vi "生成CODMn data (子VI).vi"() -> (3 "data":T1)   [LabVIEW 2016, in "斯坦道CODMn.lvlib"]
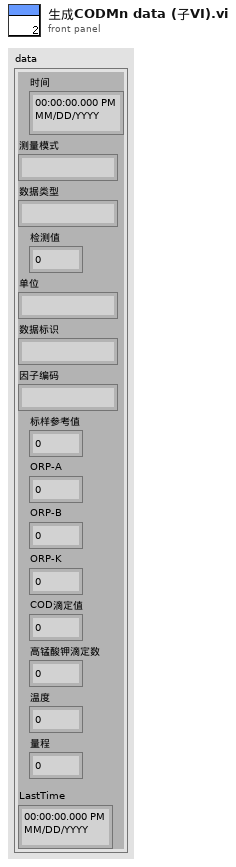
[diagram p1: front panel]
types:
  T1 = cluster{"时间":timestamp, "测量模式":string, "数据类型":string, "检测值":sgl, "单位":string, "数据标识":string, "因子编码":string, "标样参考值":sgl, "ORP-A":sgl, "ORP-B":sgl, "ORP-K":sgl, "COD滴定值":sgl, "高锰酸钾滴定数":sgl, "温度":sgl, "量程":sgl, "LastTime":timestamp}
  T2 = cluster{"运行模式":enum16{"维护模式", "常规模式", "应急模式", "质控模式"}}
  T3 = cluster{"测量量程":dbl, "测量精度":dbl, "测量间隔":dbl, "消解温度":dbl, "消解时长":dbl, "空白校准时间":timestamp, "曲线截距":dbl, "曲线斜率":dbl, "测量检出限":dbl, "测量信号值":dbl, "线性相关系数":dbl, "二次多项式系数":dbl, "标样校准时间":timestamp, "单位":u16}
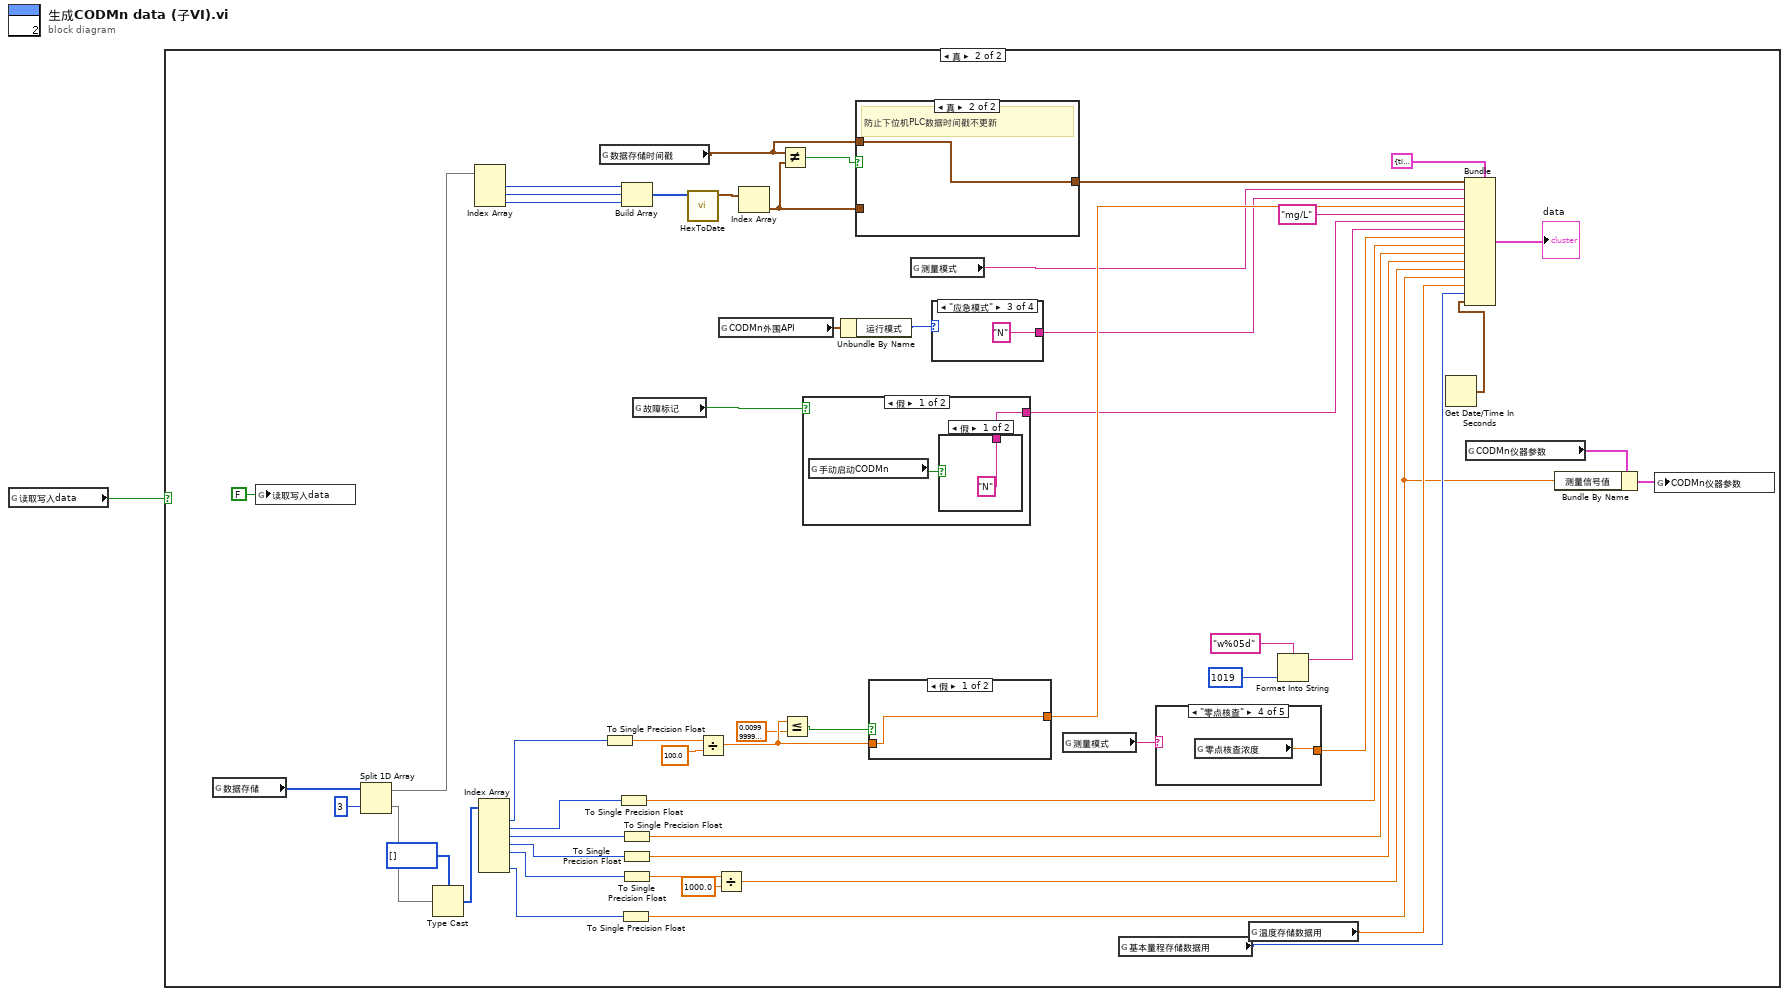
[diagram p0: block diagram]
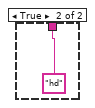
[diagram p4: hidden frame]
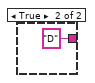
[diagram p5: hidden frame]
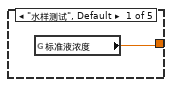
[diagram p6: hidden frame]
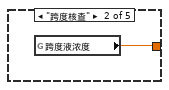
[diagram p7: hidden frame]
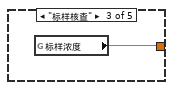
[diagram p8: hidden frame]
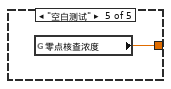
[diagram p9: hidden frame]
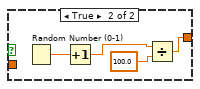
[diagram p10: hidden frame]
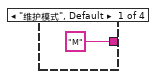
[diagram p11: hidden frame]
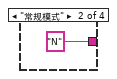
[diagram p12: hidden frame]
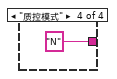
[diagram p13: hidden frame]
diagram:
  n1 = global read "COD内部交互全局.vi" "读取写入data"() -> (w1:bool)
  n2 = case shown="真" w1 {
    frame False {
    }
    frame True {
      n3 = global read "COD内部交互全局.vi" "数据存储"() -> (w7:u16[])
      n4 = global write "COD内部交互全局.vi" "读取写入data"(FALSE ("读取写入data")) -> ()
      n5 = Split 1D Array(array=w7, index=3 ("索引")) -> (first subarray=w15:u16[], second subarray=w6:u16[])
      n6 = Type Cast(type=i16[] [], x=w6) -> (*(type *) &x=w5:i16[])
      n7 = Index Array(array=w15) -> (element #1=w17:u16, element #2=w18:u16, element #3=w19:u16)  [unwired: 3 in]
      n8 = Index Array(array=w5) -> (element #1=w42:i16, element #2=w21:i16, element #3=w22:i16, element #4=w23:i16, element #5=w24:i16, element #7=w52:i16)  [unwired: 7 in, 1 out]
      n9 = global read "COD内部交互全局.vi" "数据存储时间戳"() -> (w53:timestamp)
      n10 = To Single Precision Float(number=w42) -> (single precision float=w40:sgl)
      n11 = To Single Precision Float(number=w21) -> (single precision float=w33:sgl)
      n12 = To Single Precision Float(number=w52) -> (single precision float=w2:sgl)
      n13 = Build Array(w17, w18, w19) -> (w20:u16[])
      n14 = To Single Precision Float(number=w22) -> (single precision float=w32:sgl)
      n15 = To Single Precision Float(number=w23) -> (single precision float=w31:sgl)
      n16 = To Single Precision Float(number=w24) -> (single precision float=w27:sgl)
      n17 = global read "COD内部交互全局.vi" "故障标记"() -> (w55:bool)
      n18 = call "HexToDate.vi"("数组"=w20) -> ("DATE"=w16:timestamp[])  [unwired: 10 in]
      n19 = Divide(x=w40, y=sgl 100.0) -> (x/y=w41:sgl)
      n20 = Divide(x=w27, y=sgl 1000.0) -> (x/y=w30:sgl)
      n21 = global read "CODMN外部API.vi" "CODMn外围API"() -> (w45:T2)
      n22 = Index Array(array=w16) -> (element=w48:timestamp)  [unwired: 1 in]
      n23 = Not Equal?(x=w53, y=w48) -> (x != y?=w49:bool)
      n24 = Less Or Equal?(x=w41, y=sgl 0.01) -> (x <= y?=w39:bool)
      n25 = case shown="假" w55 {
        tunnel: [w59 "D" ("数据标识")] -> w35
        frame False {
          n26 = global read "CODMN外部API.vi" "手动启动CODMn"() -> (w58:bool)
          n27 = case shown="假" w58 {
            tunnel: ["N" ("数据标识") "hd" ("数据标识")] -> w59
            frame False {
            }
            frame True {
            }
          }
        }
        frame True {
        }
      }
      n28 = Unbundle By Name(w45) -> ("运行模式"=w46:enum16{"维护模式", "常规模式", "应急模式", "质控模式"})
      n29 = case "条件结构" shown="真" w49 {
        tunnel: w48 -> [w56 _]
        tunnel: w53 -> [_ w57]
        tunnel: [w56 w57] -> w50
        frame False {
        }
        frame True {
          # "防止下位机PLC数据时间戳不更新"
        }
      }
      n30 = case shown="假" w39 {
        tunnel: [w68 w69] -> w51
        tunnel: w41 -> [w68 _]
        frame False {
        }
        frame True {
          n31 = Random Number (0-1)() -> (number: 0 to 1=w72:dbl)
          n32 = Increment(x=w72) -> (x+1=w70:dbl)
          n33 = Divide(x=w70, y=sgl 100.0) -> (x/y=w69:dbl)
        }
      }
      n34 = global read "COD测量模式全局.vi" "测量模式"() -> (w47:string)
      n35 = case shown="\"应急模式\"" w46 {
        tunnel: ["M" ("单位") "N" ("单位") "N" ("单位") "N" ("单位")] -> w37
        frame "维护模式", Default {
        }
        frame "常规模式" {
        }
        frame "应急模式" {
        }
        frame "质控模式" {
        }
      }
      n36 = global read "COD测量模式全局.vi" "测量模式"() -> (w43:string)
      n37 = global read "COD内部交互全局.vi" "基本量程存储数据用"() -> (w13:enum16{"L", "H"})
      n38 = case shown="\"零点核查\"" w43 {
        tunnel: [w63 w64 w65 w66 w67] -> w44
        frame "水样测试", Default {
          n39 = global read "COD浓度全局变量.vi" "标准液浓度"() -> (w63:dbl)
        }
        frame "跨度核查" {
          n40 = global read "CODMn断电保存全局变量.vi" "跨度液浓度"() -> (w64:dbl)
        }
        frame "标样核查" {
          n41 = global read "CODMn断电保存全局变量.vi" "标样浓度"() -> (w65:dbl)
        }
        frame "零点核查" {
          n42 = global read "CODMn断电保存全局变量.vi" "零点核查浓度"() -> (w66:dbl)
        }
        frame "空白测试" {
          n43 = global read "CODMn断电保存全局变量.vi" "零点核查浓度"() -> (w67:dbl)
        }
      }
      n44 = global read "COD内部交互全局.vi" "温度存储数据用"() -> (w54:dbl)
      n45 = Format Into String(format string="w%05d" ("格式字符串"), u32 1019 ("因子编码")) -> (resulting string=w34:string)  [unwired: 2 in, 1 out]
      n46 = Get Date/Time In Seconds() -> (seconds since 1Jan1904=w9:timestamp)
      n47 = Bundle(cluster=T1 {"时间"=timestamp(0 s since 1904-01-01), "测量模式"="", "数据类型"="", "检测值"=0.0, "单位"="", "数据标识"="", "因子编码"="", "标样参考值"=0.0, "ORP-A"=0.0, "ORP-B"=0.0, "ORP-K"=0.0, "COD滴定值"=0.0, "高锰酸钾滴定数"=0.0, "温度"=0.0, "量程"=0.0, "LastTime"=timestamp(0 s since 1904-01-01)} ("data"), "时间"=w50, "测量模式"=w47, "数据类型"=w37, "检测值"=w51, "单位"="mg/L", "数据标识"=w35, "因子编码"=w34, "标样参考值"=w44, "ORP-A"=w33, "ORP-B"=w32, "ORP-K"=w31, "COD滴定值"=w30, "高锰酸钾滴定数"=w2, "温度"=w54, "量程"=w13, "LastTime"=w9) -> (→"data":T1)
      n48 = global read "CODMn断电保存全局变量.vi" "CODMn仪器参数"() -> (w4:T3)
      n49 = Bundle By Name(cluster=w4, "测量信号值"=w2) -> (w3:T3)
      n50 = global write "CODMn断电保存全局变量.vi" "CODMn仪器参数"(w3) -> ()
    }
  }
